vi "charge amplifier.vi"() -> ()   [LabVIEW 2020]
uses:
  <vilib>/Instr/_visa.llb/VISA Configure Serial Port (Instr).vi
panel:
  out "LED CH 4":bool
  out "LED CH 3":bool
  out "LED CH 2":bool
  out "LED CH 1":bool
  in  "CHANNEL 4":bool
  in  "CHANNEL 3":bool
  in  "CHANNEL 2":bool
  in  "CHANNEL 1":bool
  out "Array":bool[](array[boolean])
  in  "ENABLE":bool
  in  "stop":bool
  in  "VISA resource (Arduino)":refnum<visa-resource-name>
  in  "Write":string
  in  "GA2 7":bool
  in  "GA2 6":bool
  in  "GA2 5":bool
  in  "GA2 4":bool
  in  "GA2 3":bool
  in  "GA2 2":bool
  in  "GA2 1":bool
  in  "GA2 0":bool
  in  "GA1 7":bool
  in  "GA1 6":bool
  in  "GA1 5":bool
  in  "GA1 4":bool
  in  "GA1 3":bool
  in  "GA1 2":bool
  in  "GA1 1":bool
  in  "GA1 0":bool
  in  "MUX2 7":bool
  in  "MUX2 6":bool
  in  "MUX2 5":bool
  in  "MUX2 4":bool
  in  "MUX2 3":bool
  in  "MUX2 2":bool
  in  "MUX2 1":bool
  in  "MUX2 0":bool
  in  "MUX1 7":bool
  in  "MUX1 6":bool
  in  "MUX1 5":bool
  in  "MUX1 4":bool
  in  "MUX1 3":bool
  in  "MUX1 2":bool
  in  "MUX1 1":bool
  in  "MUX1 0":bool
  in  "EM2 0":bool
  in  "EM2 1":bool
  in  "EM1 0":bool
  in  "EM1 1":bool
  # "EM1"
  # "EM2"
  # "MUX1"
  # "MUX2"
  # "GAIN1"
  # "GAIN1"
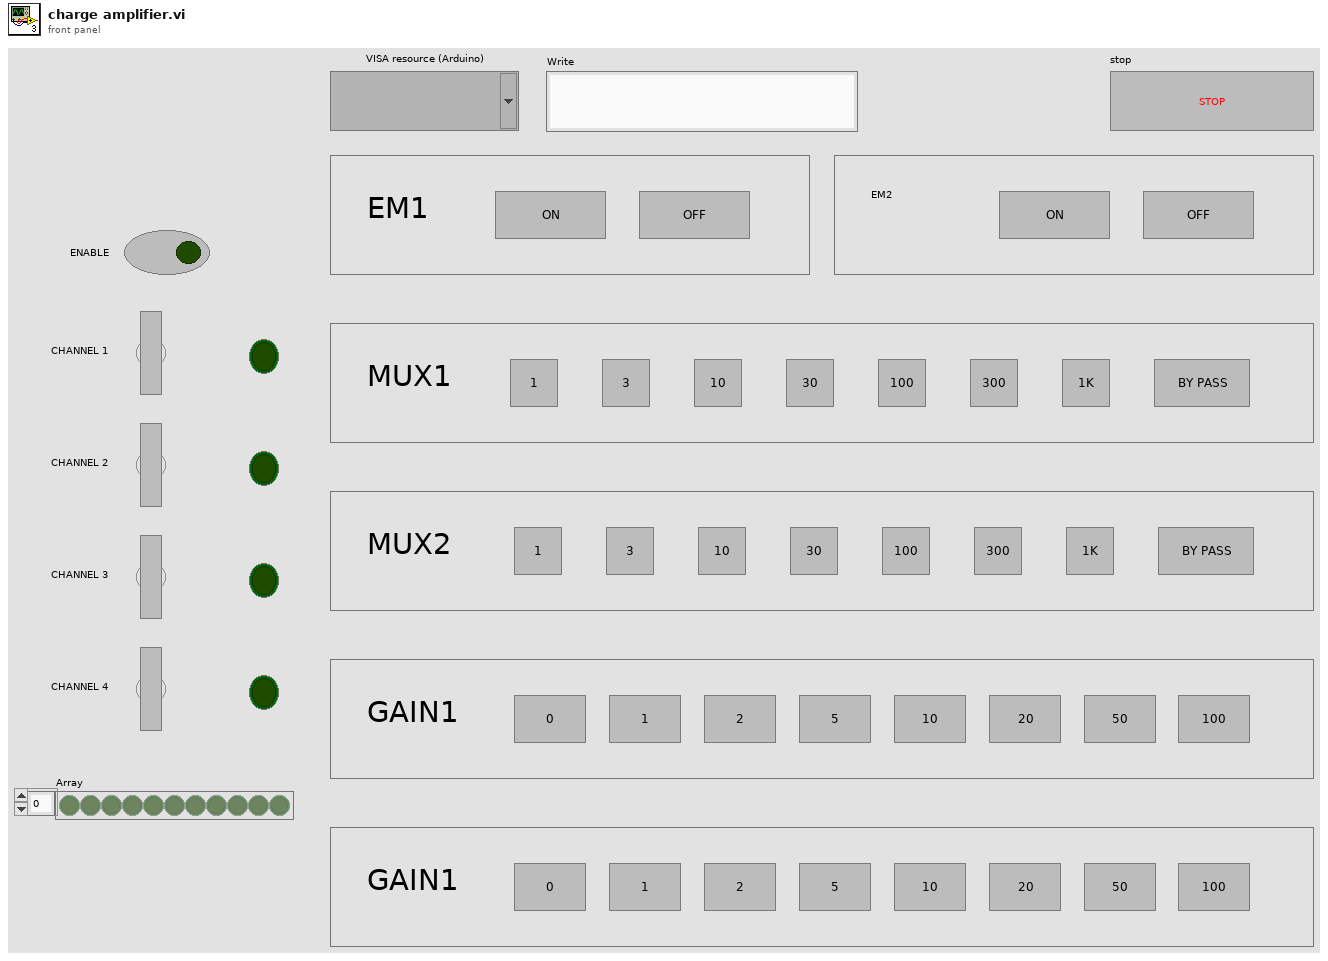
[diagram p1: front panel]
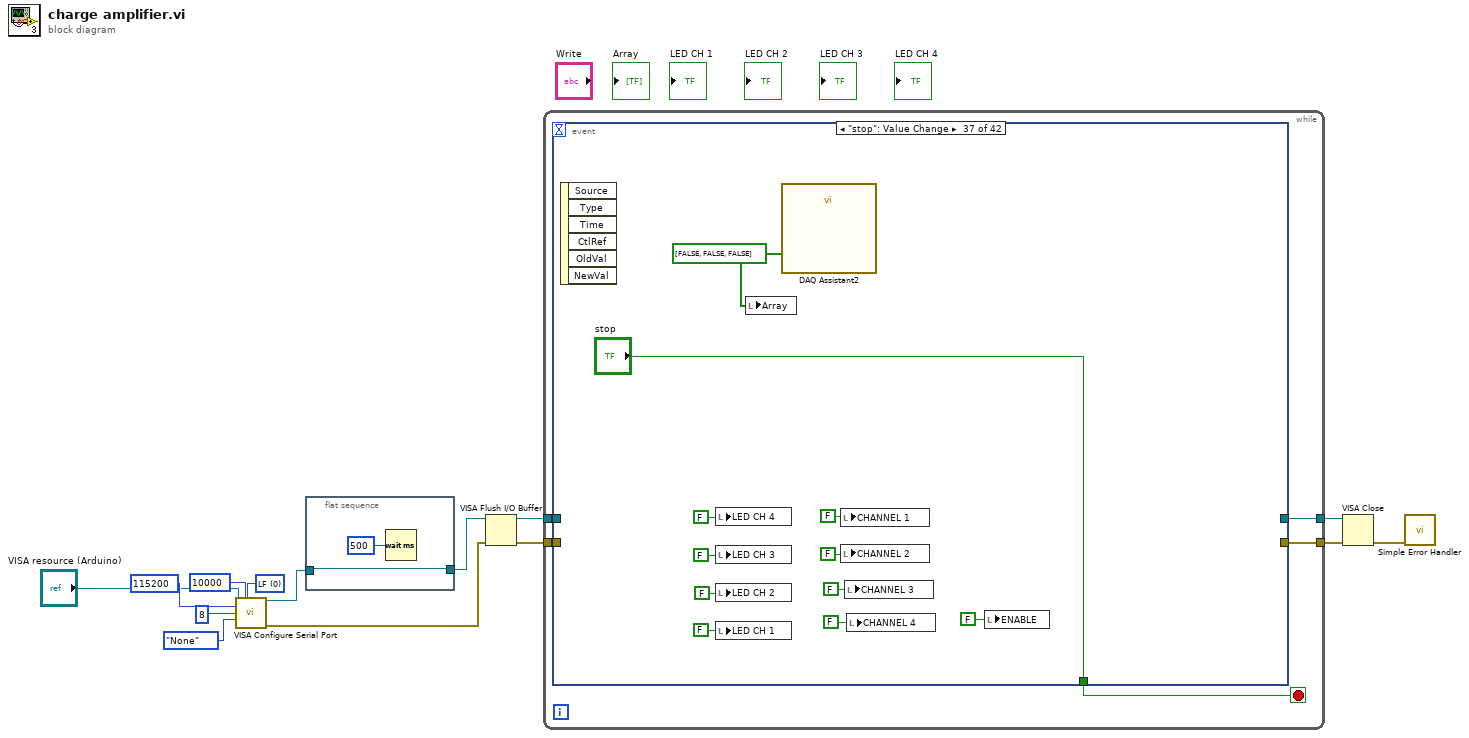
[diagram p0: block diagram]
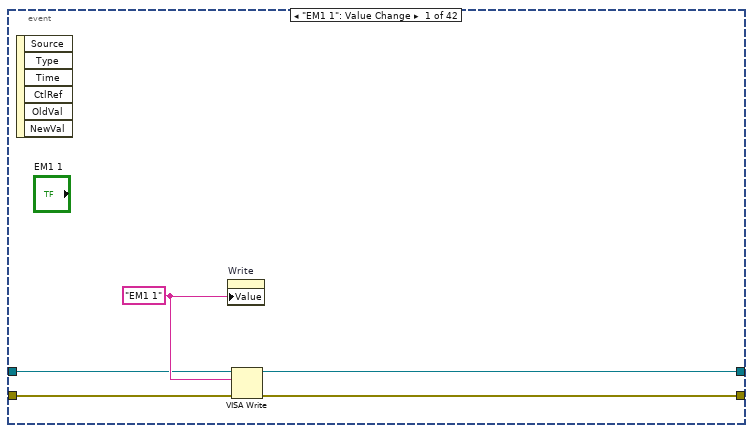
[diagram p2: hidden frame]
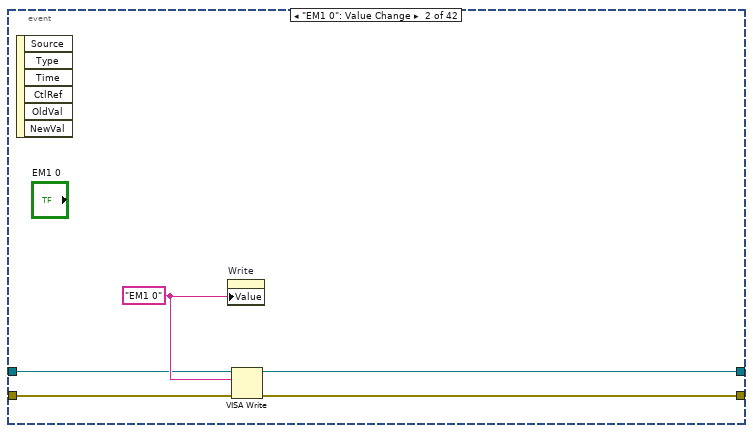
[diagram p3: hidden frame]
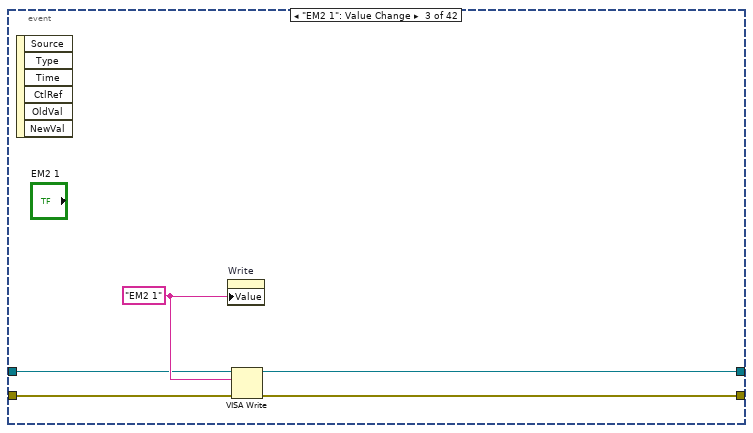
[diagram p4: hidden frame]
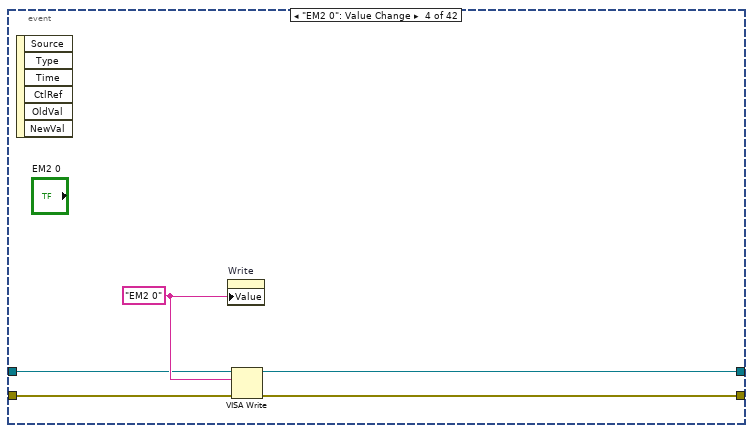
[diagram p5: hidden frame]
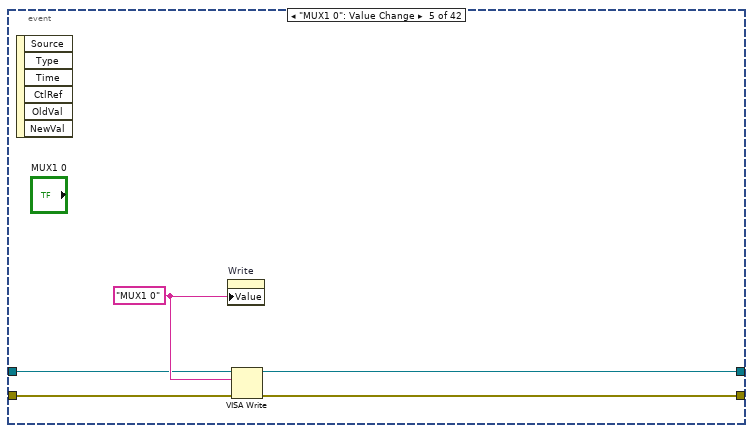
[diagram p6: hidden frame]
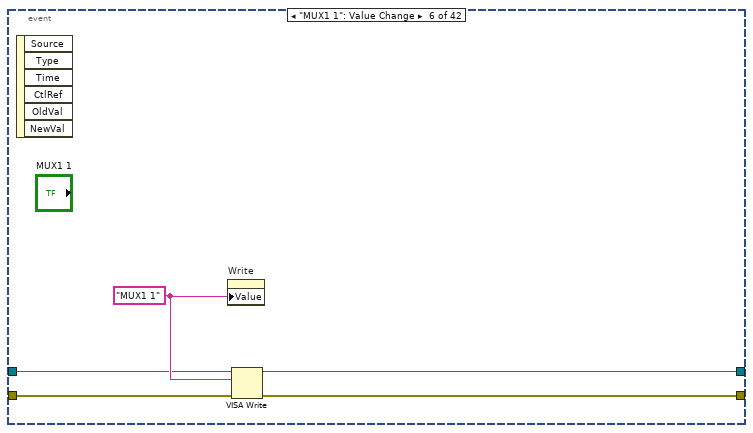
[diagram p7: hidden frame]
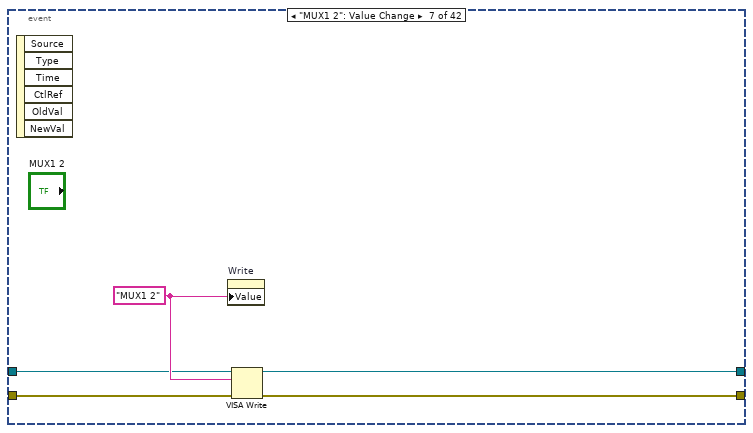
[diagram p8: hidden frame]
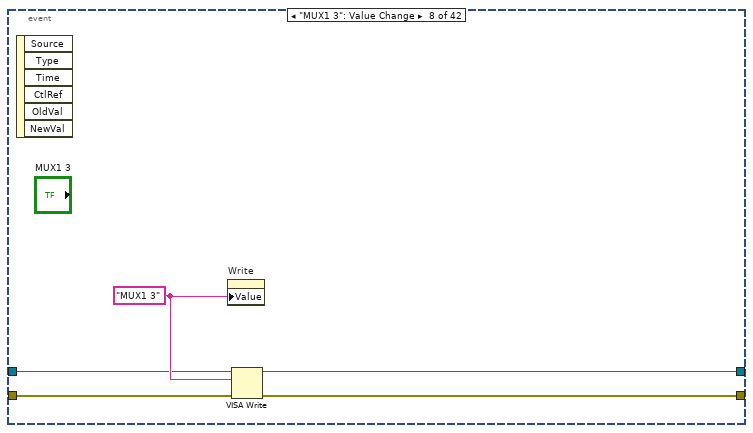
[diagram p9: hidden frame]
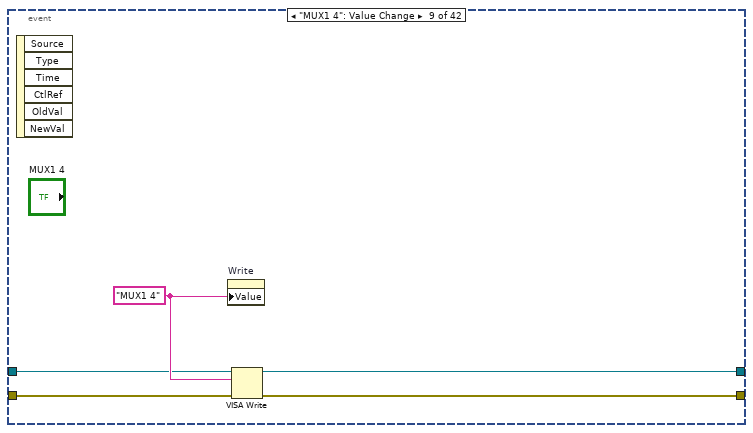
[diagram p10: hidden frame]
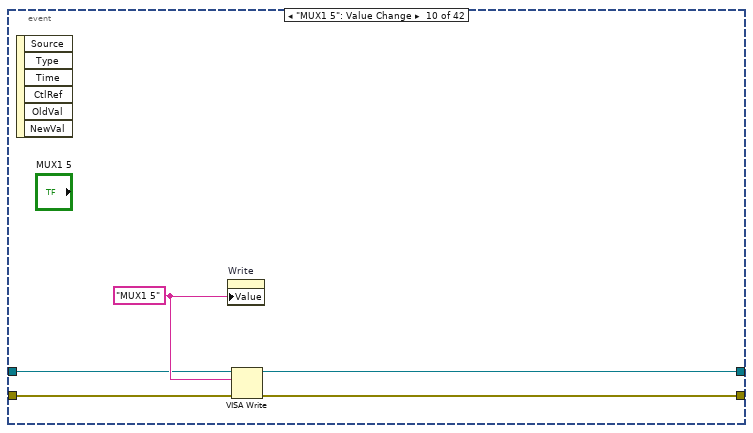
[diagram p11: hidden frame]
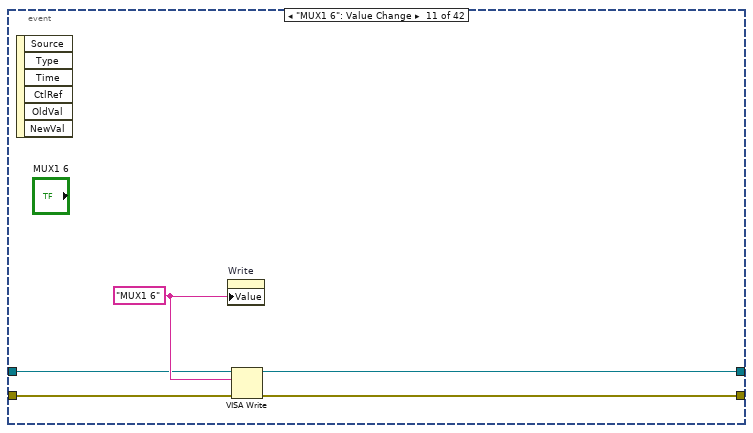
[diagram p12: hidden frame]
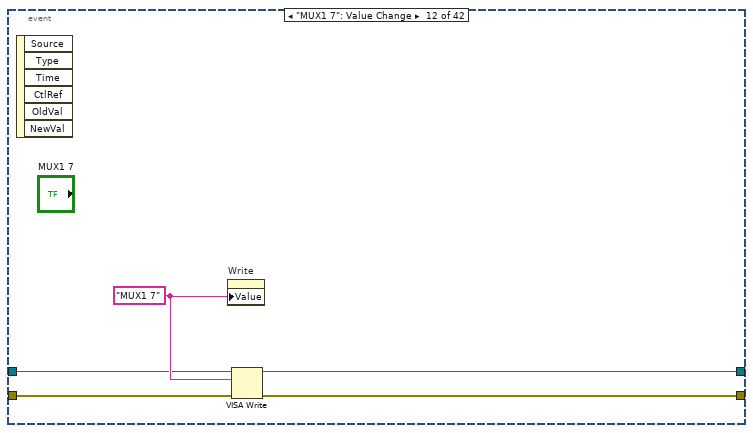
[diagram p13: hidden frame]
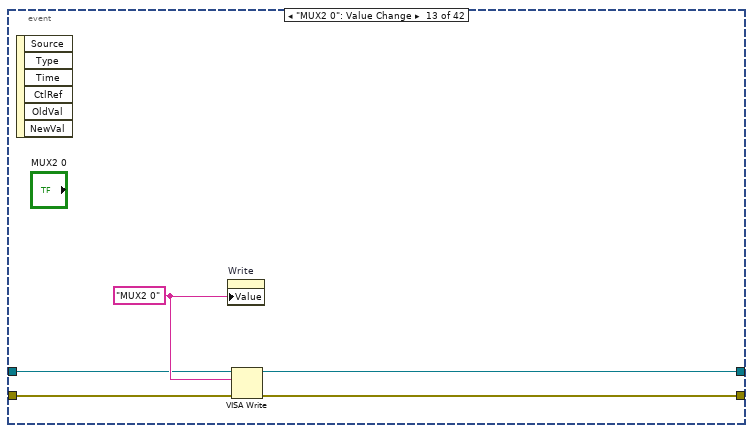
[diagram p14: hidden frame]
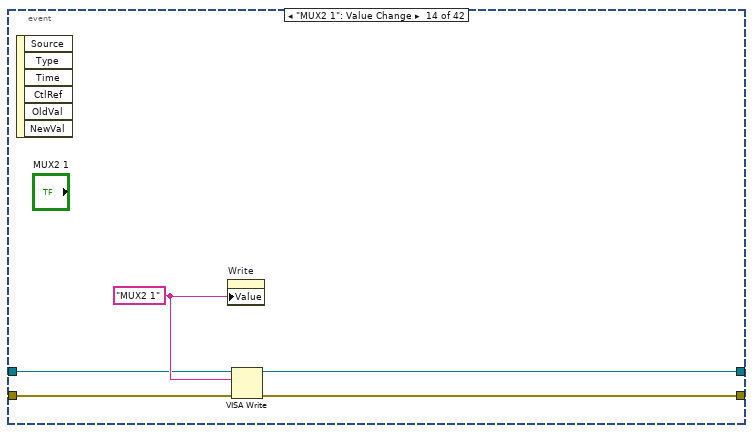
[diagram p15: hidden frame]
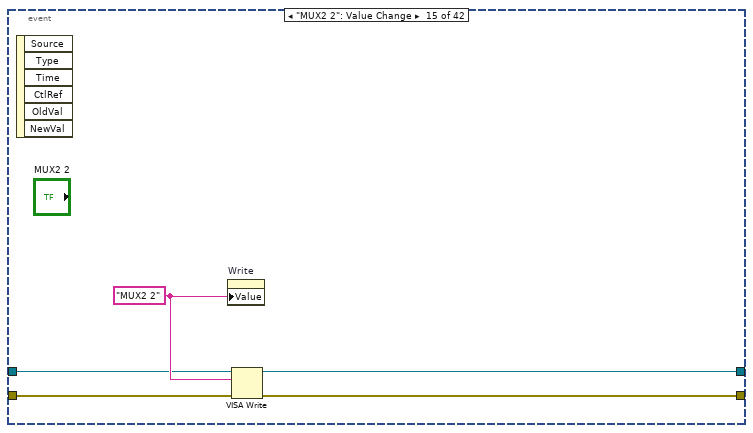
[diagram p16: hidden frame]
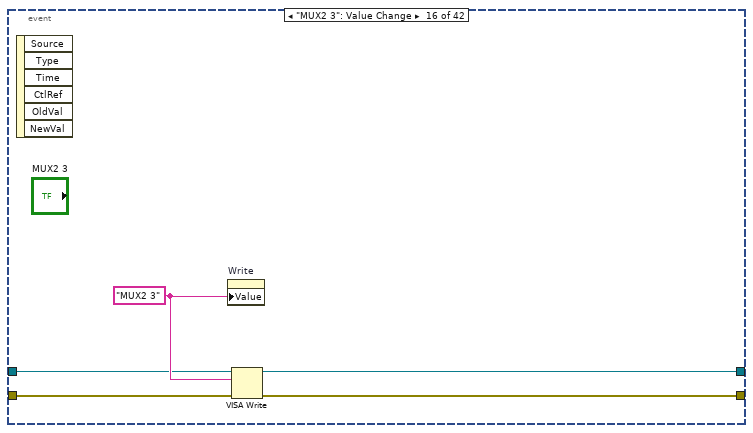
[diagram p17: hidden frame]
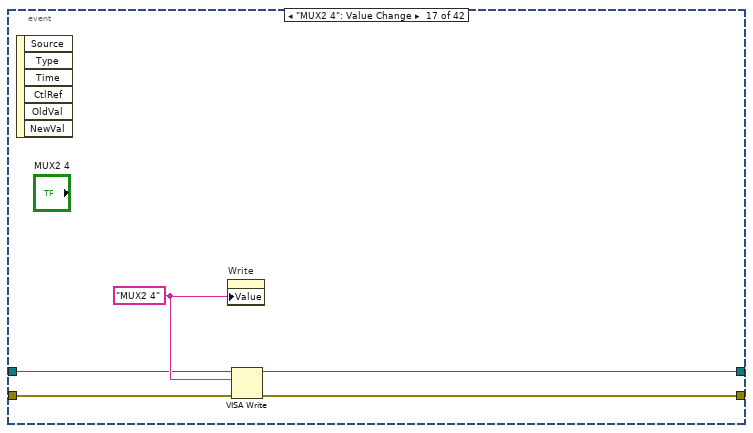
[diagram p18: hidden frame]
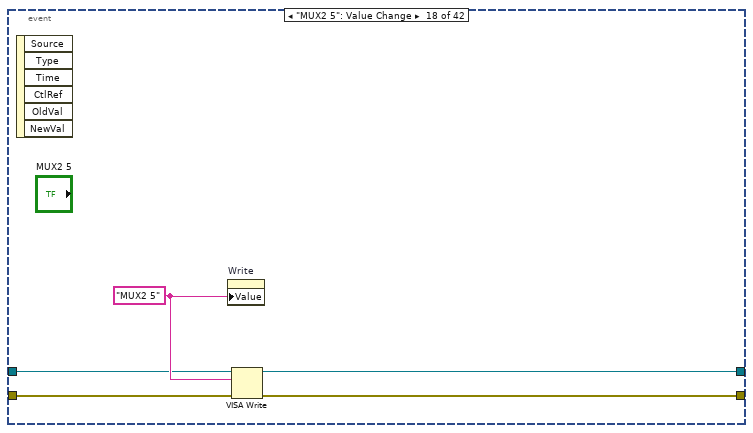
[diagram p19: hidden frame]
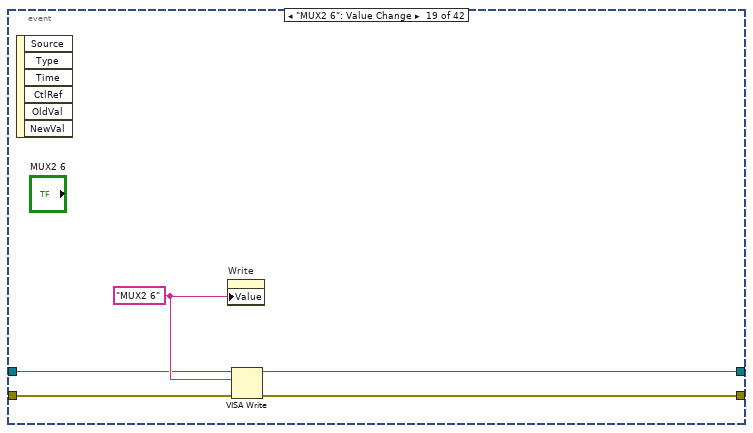
[diagram p20: hidden frame]
diagram:
  w11 = u16 0 items=["LF"]
  n1 = call-poly "VISA Configure Serial Port"("VISA resource name"="VISA resource (Arduino)", "timeout (10sec)"=u32 10000, "termination char\n(0xA = '\\n' = LF)"=w11, "baud rate (9600)"=u32 115200, "data bits (8)"=u16 8, "parity (0:none)"=enum16{"None", "Odd", "Even", "Mark", "Space"}."None") -> ("VISA resource name out"=w7:refnum<visa-resource-name>, "error out"=w5:errorcluster)  [unwired: 8 in]
  n2 = flat-sequence {
    tunnel: [w15] -> w6
    tunnel: w7 -> [w15]
    frame #0 {
      n3 = Wait (ms)(milliseconds to wait=u32 500 ("대기 시간(ms)")) -> ()  [unwired: 1 out]
    }
  }
  n4 = VISA Flush I/O Buffer(VISA resource name=w6, error in (no error)=w5) -> (VISA resource name out=w3:refnum<visa-resource-name>, error out=w2:errorcluster)  [unwired: 1 in]
  n5 = while {
    tunnel: w3 -> [w21]
    tunnel: w2 -> [w20]
    tunnel: [w19] -> w14
    tunnel: [w18] -> w13
    stop <- w17 stop-if-true
    n6 = event shown="[36] \"stop\": Value Change" {
      selector: _ -> [_ _ _ _ _ _ _ _ _ _ _ _ _ _ _ _ _ _ _ _ _ _ _ _ _ _ _ _ _ _ _ _ _ _ _ _ _ _ _ _ _ _]
      dyn-events: _ -> [_ _ _ _ _ _ _ _ _ _ _ _ _ _ _ _ _ _ _ _ _ _ _ _ _ _ _ _ _ _ _ _ _ _ _ _ _ _ _ _ _ _]
      timeout: _ -> [_ _ _ _ _ _ _ _ _ _ _ _ _ _ _ _ _ _ _ _ _ _ _ _ _ _ _ _ _ _ _ _ _ _ _ _ _ _ _ _ _ _]
      tunnel: w21 -> [w25 w30 w35 w40 w45 w50 w55 w60 w65 w70 w75 w80 w85 w90 w95 w100 w105 w110 w115 w120 w125 w130 w135 w140 w145 w150 w155 w160 w165 w170 w175 w180 w185 w190 w195 w200 _ _ _ _ _ _]
      tunnel: w20 -> [w24 w29 w34 w39 w44 w49 w54 w59 w64 w69 w74 w79 w84 w89 w94 w99 w104 w109 w114 w119 w124 w129 w134 w139 w144 w149 w154 w159 w164 w169 w174 w179 w184 w189 w194 w199 _ _ _ _ _ _]
      tunnel: [w23 w28 w33 w38 w43 w48 w53 w58 w63 w68 w73 w78 w83 w88 w93 w98 w103 w108 w113 w118 w123 w128 w133 w138 w143 w148 w153 w158 w163 w168 w173 w178 w183 w188 w193 w198 _ _ _ _ _ _] -> w19
      tunnel: [w22 w27 w32 w37 w42 w47 w52 w57 w62 w67 w72 w77 w82 w87 w92 w97 w102 w107 w112 w117 w122 w127 w132 w137 w142 w147 w152 w157 w162 w167 w172 w177 w182 w187 w192 w197 _ _ _ _ _ _] -> w18
      tunnel: [_ _ _ _ _ _ _ _ _ _ _ _ _ _ _ _ _ _ _ _ _ _ _ _ _ _ _ _ _ _ _ _ _ _ _ _ "stop" _ _ _ _ _] -> w17
      event "EM1 1": Value Change {
        w26 = "EM1 1" ("Write")
        n7 = event-data() -> ()  [unwired: 1 in, 6 out]
        n8 = property on="Write" class="Str"("Value"=w26) -> ()  [unwired: 2 in, 2 out]
        n9 = VISA Write(VISA resource name=w25, write buffer=w26, error in (no error)=w24) -> (VISA resource name out=w23:refnum<visa-resource-name>, error out=w22:errorcluster)  [unwired: 1 out]
      }
      event "EM1 0": Value Change {
        w31 = "EM1 0" ("Write")
        n10 = event-data() -> ()  [unwired: 1 in, 6 out]
        n11 = property on="Write" class="Str"("Value"=w31) -> ()  [unwired: 2 in, 2 out]
        n12 = VISA Write(VISA resource name=w30, write buffer=w31, error in (no error)=w29) -> (VISA resource name out=w28:refnum<visa-resource-name>, error out=w27:errorcluster)  [unwired: 1 out]
      }
      event "EM2 1": Value Change {
        w36 = "EM2 1" ("Write")
        n13 = event-data() -> ()  [unwired: 1 in, 6 out]
        n14 = property on="Write" class="Str"("Value"=w36) -> ()  [unwired: 2 in, 2 out]
        n15 = VISA Write(VISA resource name=w35, write buffer=w36, error in (no error)=w34) -> (VISA resource name out=w33:refnum<visa-resource-name>, error out=w32:errorcluster)  [unwired: 1 out]
      }
      event "EM2 0": Value Change {
        w41 = "EM2 0" ("Write")
        n16 = event-data() -> ()  [unwired: 1 in, 6 out]
        n17 = property on="Write" class="Str"("Value"=w41) -> ()  [unwired: 2 in, 2 out]
        n18 = VISA Write(VISA resource name=w40, write buffer=w41, error in (no error)=w39) -> (VISA resource name out=w38:refnum<visa-resource-name>, error out=w37:errorcluster)  [unwired: 1 out]
      }
      event "MUX1 0": Value Change {
        w46 = "MUX1 0" ("Write")
        n19 = event-data() -> ()  [unwired: 1 in, 6 out]
        n20 = property on="Write" class="Str"("Value"=w46) -> ()  [unwired: 2 in, 2 out]
        n21 = VISA Write(VISA resource name=w45, write buffer=w46, error in (no error)=w44) -> (VISA resource name out=w43:refnum<visa-resource-name>, error out=w42:errorcluster)  [unwired: 1 out]
      }
      event "MUX1 1": Value Change {
        w51 = "MUX1 1" ("Write")
        n22 = event-data() -> ()  [unwired: 1 in, 6 out]
        n23 = property on="Write" class="Str"("Value"=w51) -> ()  [unwired: 2 in, 2 out]
        n24 = VISA Write(VISA resource name=w50, write buffer=w51, error in (no error)=w49) -> (VISA resource name out=w48:refnum<visa-resource-name>, error out=w47:errorcluster)  [unwired: 1 out]
      }
      event "MUX1 2": Value Change {
        w56 = "MUX1 2" ("Write")
        n25 = event-data() -> ()  [unwired: 1 in, 6 out]
        n26 = property on="Write" class="Str"("Value"=w56) -> ()  [unwired: 2 in, 2 out]
        n27 = VISA Write(VISA resource name=w55, write buffer=w56, error in (no error)=w54) -> (VISA resource name out=w53:refnum<visa-resource-name>, error out=w52:errorcluster)  [unwired: 1 out]
      }
      event "MUX1 3": Value Change {
        w61 = "MUX1 3" ("Write")
        n28 = event-data() -> ()  [unwired: 1 in, 6 out]
        n29 = property on="Write" class="Str"("Value"=w61) -> ()  [unwired: 2 in, 2 out]
        n30 = VISA Write(VISA resource name=w60, write buffer=w61, error in (no error)=w59) -> (VISA resource name out=w58:refnum<visa-resource-name>, error out=w57:errorcluster)  [unwired: 1 out]
      }
      event "MUX1 4": Value Change {
        w66 = "MUX1 4" ("Write")
        n31 = event-data() -> ()  [unwired: 1 in, 6 out]
        n32 = property on="Write" class="Str"("Value"=w66) -> ()  [unwired: 2 in, 2 out]
        n33 = VISA Write(VISA resource name=w65, write buffer=w66, error in (no error)=w64) -> (VISA resource name out=w63:refnum<visa-resource-name>, error out=w62:errorcluster)  [unwired: 1 out]
      }
      event "MUX1 5": Value Change {
        w71 = "MUX1 5" ("Write")
        n34 = event-data() -> ()  [unwired: 1 in, 6 out]
        n35 = property on="Write" class="Str"("Value"=w71) -> ()  [unwired: 2 in, 2 out]
        n36 = VISA Write(VISA resource name=w70, write buffer=w71, error in (no error)=w69) -> (VISA resource name out=w68:refnum<visa-resource-name>, error out=w67:errorcluster)  [unwired: 1 out]
      }
      event "MUX1 6": Value Change {
        w76 = "MUX1 6" ("Write")
        n37 = event-data() -> ()  [unwired: 1 in, 6 out]
        n38 = property on="Write" class="Str"("Value"=w76) -> ()  [unwired: 2 in, 2 out]
        n39 = VISA Write(VISA resource name=w75, write buffer=w76, error in (no error)=w74) -> (VISA resource name out=w73:refnum<visa-resource-name>, error out=w72:errorcluster)  [unwired: 1 out]
      }
      event "MUX1 7": Value Change {
        w81 = "MUX1 7" ("Write")
        n40 = event-data() -> ()  [unwired: 1 in, 6 out]
        n41 = property on="Write" class="Str"("Value"=w81) -> ()  [unwired: 2 in, 2 out]
        n42 = VISA Write(VISA resource name=w80, write buffer=w81, error in (no error)=w79) -> (VISA resource name out=w78:refnum<visa-resource-name>, error out=w77:errorcluster)  [unwired: 1 out]
      }
      event "MUX2 0": Value Change {
        w86 = "MUX2 0" ("Write")
        n43 = event-data() -> ()  [unwired: 1 in, 6 out]
        n44 = property on="Write" class="Str"("Value"=w86) -> ()  [unwired: 2 in, 2 out]
        n45 = VISA Write(VISA resource name=w85, write buffer=w86, error in (no error)=w84) -> (VISA resource name out=w83:refnum<visa-resource-name>, error out=w82:errorcluster)  [unwired: 1 out]
      }
      event "MUX2 1": Value Change {
        w91 = "MUX2 1" ("Write")
        n46 = event-data() -> ()  [unwired: 1 in, 6 out]
        n47 = property on="Write" class="Str"("Value"=w91) -> ()  [unwired: 2 in, 2 out]
        n48 = VISA Write(VISA resource name=w90, write buffer=w91, error in (no error)=w89) -> (VISA resource name out=w88:refnum<visa-resource-name>, error out=w87:errorcluster)  [unwired: 1 out]
      }
      event "MUX2 2": Value Change {
        w96 = "MUX2 2" ("Write")
        n49 = event-data() -> ()  [unwired: 1 in, 6 out]
        n50 = property on="Write" class="Str"("Value"=w96) -> ()  [unwired: 2 in, 2 out]
        n51 = VISA Write(VISA resource name=w95, write buffer=w96, error in (no error)=w94) -> (VISA resource name out=w93:refnum<visa-resource-name>, error out=w92:errorcluster)  [unwired: 1 out]
      }
      event "MUX2 3": Value Change {
        w101 = "MUX2 3" ("Write")
        n52 = event-data() -> ()  [unwired: 1 in, 6 out]
        n53 = property on="Write" class="Str"("Value"=w101) -> ()  [unwired: 2 in, 2 out]
        n54 = VISA Write(VISA resource name=w100, write buffer=w101, error in (no error)=w99) -> (VISA resource name out=w98:refnum<visa-resource-name>, error out=w97:errorcluster)  [unwired: 1 out]
      }
      event "MUX2 4": Value Change {
        w106 = "MUX2 4" ("Write")
        n55 = event-data() -> ()  [unwired: 1 in, 6 out]
        n56 = property on="Write" class="Str"("Value"=w106) -> ()  [unwired: 2 in, 2 out]
        n57 = VISA Write(VISA resource name=w105, write buffer=w106, error in (no error)=w104) -> (VISA resource name out=w103:refnum<visa-resource-name>, error out=w102:errorcluster)  [unwired: 1 out]
      }
      event "MUX2 5": Value Change {
        w111 = "MUX2 5" ("Write")
        n58 = event-data() -> ()  [unwired: 1 in, 6 out]
        n59 = property on="Write" class="Str"("Value"=w111) -> ()  [unwired: 2 in, 2 out]
        n60 = VISA Write(VISA resource name=w110, write buffer=w111, error in (no error)=w109) -> (VISA resource name out=w108:refnum<visa-resource-name>, error out=w107:errorcluster)  [unwired: 1 out]
      }
      event "MUX2 6": Value Change {
        w116 = "MUX2 6" ("Write")
        n61 = event-data() -> ()  [unwired: 1 in, 6 out]
        n62 = property on="Write" class="Str"("Value"=w116) -> ()  [unwired: 2 in, 2 out]
        n63 = VISA Write(VISA resource name=w115, write buffer=w116, error in (no error)=w114) -> (VISA resource name out=w113:refnum<visa-resource-name>, error out=w112:errorcluster)  [unwired: 1 out]
      }
      event "MUX2 7": Value Change {
        w121 = "MUX2 7" ("Write")
        n64 = event-data() -> ()  [unwired: 1 in, 6 out]
        n65 = property on="Write" class="Str"("Value"=w121) -> ()  [unwired: 2 in, 2 out]
        n66 = VISA Write(VISA resource name=w120, write buffer=w121, error in (no error)=w119) -> (VISA resource name out=w118:refnum<visa-resource-name>, error out=w117:errorcluster)  [unwired: 1 out]
      }
      event "GA1 0": Value Change {
        w126 = "GA1 0" ("Write")
        n67 = event-data() -> ()  [unwired: 1 in, 6 out]
        n68 = property on="Write" class="Str"("Value"=w126) -> ()  [unwired: 2 in, 2 out]
        n69 = VISA Write(VISA resource name=w125, write buffer=w126, error in (no error)=w124) -> (VISA resource name out=w123:refnum<visa-resource-name>, error out=w122:errorcluster)  [unwired: 1 out]
      }
      event "GA1 1": Value Change {
        w131 = "GA1 1" ("Write")
        n70 = event-data() -> ()  [unwired: 1 in, 6 out]
        n71 = property on="Write" class="Str"("Value"=w131) -> ()  [unwired: 2 in, 2 out]
        n72 = VISA Write(VISA resource name=w130, write buffer=w131, error in (no error)=w129) -> (VISA resource name out=w128:refnum<visa-resource-name>, error out=w127:errorcluster)  [unwired: 1 out]
      }
      event "GA1 2": Value Change {
        w136 = "GA1 2" ("Write")
        n73 = event-data() -> ()  [unwired: 1 in, 6 out]
        n74 = property on="Write" class="Str"("Value"=w136) -> ()  [unwired: 2 in, 2 out]
        n75 = VISA Write(VISA resource name=w135, write buffer=w136, error in (no error)=w134) -> (VISA resource name out=w133:refnum<visa-resource-name>, error out=w132:errorcluster)  [unwired: 1 out]
      }
      event "GA1 3": Value Change {
        w141 = "GA1 3" ("Write")
        n76 = event-data() -> ()  [unwired: 1 in, 6 out]
        n77 = property on="Write" class="Str"("Value"=w141) -> ()  [unwired: 2 in, 2 out]
        n78 = VISA Write(VISA resource name=w140, write buffer=w141, error in (no error)=w139) -> (VISA resource name out=w138:refnum<visa-resource-name>, error out=w137:errorcluster)  [unwired: 1 out]
      }
      event "GA1 4": Value Change {
        w146 = "GA1 4" ("Write")
        n79 = event-data() -> ()  [unwired: 1 in, 6 out]
        n80 = property on="Write" class="Str"("Value"=w146) -> ()  [unwired: 2 in, 2 out]
        n81 = VISA Write(VISA resource name=w145, write buffer=w146, error in (no error)=w144) -> (VISA resource name out=w143:refnum<visa-resource-name>, error out=w142:errorcluster)  [unwired: 1 out]
      }
      event "GA1 5": Value Change {
        w151 = "GA1 5" ("Write")
        n82 = event-data() -> ()  [unwired: 1 in, 6 out]
        n83 = property on="Write" class="Str"("Value"=w151) -> ()  [unwired: 2 in, 2 out]
        n84 = VISA Write(VISA resource name=w150, write buffer=w151, error in (no error)=w149) -> (VISA resource name out=w148:refnum<visa-resource-name>, error out=w147:errorcluster)  [unwired: 1 out]
      }
      event "GA1 6": Value Change {
        w156 = "GA1 6" ("Write")
        n85 = event-data() -> ()  [unwired: 1 in, 6 out]
        n86 = property on="Write" class="Str"("Value"=w156) -> ()  [unwired: 2 in, 2 out]
        n87 = VISA Write(VISA resource name=w155, write buffer=w156, error in (no error)=w154) -> (VISA resource name out=w153:refnum<visa-resource-name>, error out=w152:errorcluster)  [unwired: 1 out]
      }
      event "GA1 7": Value Change {
        w161 = "GA1 7" ("Write")
        n88 = event-data() -> ()  [unwired: 1 in, 6 out]
        n89 = property on="Write" class="Str"("Value"=w161) -> ()  [unwired: 2 in, 2 out]
        n90 = VISA Write(VISA resource name=w160, write buffer=w161, error in (no error)=w159) -> (VISA resource name out=w158:refnum<visa-resource-name>, error out=w157:errorcluster)  [unwired: 1 out]
      }
      event "GA2 0": Value Change {
        w166 = "GA2 0" ("Write")
        n91 = event-data() -> ()  [unwired: 1 in, 6 out]
        n92 = property on="Write" class="Str"("Value"=w166) -> ()  [unwired: 2 in, 2 out]
        n93 = VISA Write(VISA resource name=w165, write buffer=w166, error in (no error)=w164) -> (VISA resource name out=w163:refnum<visa-resource-name>, error out=w162:errorcluster)  [unwired: 1 out]
      }
      event "GA2 1": Value Change {
        w171 = "GA2 1" ("Write")
        n94 = event-data() -> ()  [unwired: 1 in, 6 out]
        n95 = property on="Write" class="Str"("Value"=w171) -> ()  [unwired: 2 in, 2 out]
        n96 = VISA Write(VISA resource name=w170, write buffer=w171, error in (no error)=w169) -> (VISA resource name out=w168:refnum<visa-resource-name>, error out=w167:errorcluster)  [unwired: 1 out]
      }
      event "GA2 2": Value Change {
        w176 = "GA2 2" ("Write")
        n97 = event-data() -> ()  [unwired: 1 in, 6 out]
        n98 = property on="Write" class="Str"("Value"=w176) -> ()  [unwired: 2 in, 2 out]
        n99 = VISA Write(VISA resource name=w175, write buffer=w176, error in (no error)=w174) -> (VISA resource name out=w173:refnum<visa-resource-name>, error out=w172:errorcluster)  [unwired: 1 out]
      }
      event "GA2 3": Value Change {
        w181 = "GA2 3" ("Write")
        n100 = event-data() -> ()  [unwired: 1 in, 6 out]
        n101 = property on="Write" class="Str"("Value"=w181) -> ()  [unwired: 2 in, 2 out]
        n102 = VISA Write(VISA resource name=w180, write buffer=w181, error in (no error)=w179) -> (VISA resource name out=w178:refnum<visa-resource-name>, error out=w177:errorcluster)  [unwired: 1 out]
      }
      event "GA2 4": Value Change {
        w186 = "GA2 4" ("Write")
        n103 = event-data() -> ()  [unwired: 1 in, 6 out]
        n104 = property on="Write" class="Str"("Value"=w186) -> ()  [unwired: 2 in, 2 out]
        n105 = VISA Write(VISA resource name=w185, write buffer=w186, error in (no error)=w184) -> (VISA resource name out=w183:refnum<visa-resource-name>, error out=w182:errorcluster)  [unwired: 1 out]
      }
      event "GA2 5": Value Change {
        w191 = "GA2 5" ("Write")
        n106 = event-data() -> ()  [unwired: 1 in, 6 out]
        n107 = property on="Write" class="Str"("Value"=w191) -> ()  [unwired: 2 in, 2 out]
        n108 = VISA Write(VISA resource name=w190, write buffer=w191, error in (no error)=w189) -> (VISA resource name out=w188:refnum<visa-resource-name>, error out=w187:errorcluster)  [unwired: 1 out]
      }
      event "GA2 6": Value Change {
        w196 = "GA2 6" ("Write")
        n109 = event-data() -> ()  [unwired: 1 in, 6 out]
        n110 = property on="Write" class="Str"("Value"=w196) -> ()  [unwired: 2 in, 2 out]
        n111 = VISA Write(VISA resource name=w195, write buffer=w196, error in (no error)=w194) -> (VISA resource name out=w193:refnum<visa-resource-name>, error out=w192:errorcluster)  [unwired: 1 out]
      }
      event "GA2 7": Value Change {
        w201 = "GA2 7" ("Write")
        n112 = event-data() -> ()  [unwired: 1 in, 6 out]
        n113 = property on="Write" class="Str"("Value"=w201) -> ()  [unwired: 2 in, 2 out]
        n114 = VISA Write(VISA resource name=w200, write buffer=w201, error in (no error)=w199) -> (VISA resource name out=w198:refnum<visa-resource-name>, error out=w197:errorcluster)  [unwired: 1 out]
      }
      event "stop": Value Change {
        w202 = bool[] [FALSE, FALSE, FALSE]
        n115 = event-data() -> ()  [unwired: 1 in, 6 out]
        n116 = local write "LED CH 4"(FALSE ("ENABLE")) -> ()
        n117 = local write "LED CH 3"(FALSE ("ENABLE")) -> ()
        n118 = local write "LED CH 2"(FALSE ("ENABLE")) -> ()
        n119 = local write "LED CH 1"(FALSE ("ENABLE")) -> ()
        n120 = local write "Array"(w202) -> ()
        n121 = call "DAQ Assistant2"("data"=w202) -> ()  [unwired: 17 in, 2 out]
        n122 = local write "CHANNEL 1"(FALSE ("ENABLE")) -> ()
        n123 = local write "CHANNEL 2"(FALSE ("ENABLE")) -> ()
        n124 = local write "CHANNEL 3"(FALSE ("ENABLE")) -> ()
        n125 = local write "CHANNEL 4"(FALSE ("ENABLE")) -> ()
        n126 = local write "ENABLE"(FALSE ("ENABLE")) -> ()
      }
      event "CHANNEL 1": Value Change {
        n127 = event-data() -> ()  [unwired: 1 in, 6 out]
        n128 = local read "ENABLE"() -> (w213:bool)
        n129 = case shown="True" w213 {
          frame False {
          }
          frame True {
            w215 = FALSE ("CHANNEL 4")
            w216 = FALSE ("CHANNEL 3")
            w217 = FALSE ("CHANNEL 2")
            w218 = bool[] [TRUE, FALSE, FALSE]
            n130 = property on="CHANNEL 3" class="Bool (strict)"("Value"=w216) -> ()  [unwired: 2 in, 2 out]
            n131 = property on="CHANNEL 2" class="Bool (strict)"("Value"=w217) -> ()  [unwired: 2 in, 2 out]
            n132 = property on="CHANNEL 4" class="Bool (strict)"("Value"=w215) -> ()  [unwired: 2 in, 2 out]
            n133 = local write "LED CH 1"(TRUE ("LED CH 1")) -> ()
            n134 = local write "LED CH 2"(w217) -> ()
            n135 = local write "LED CH 3"(w216) -> ()
            n136 = local write "LED CH 4"(w215) -> ()
            n137 = local write "Array"(w218) -> ()
            n138 = call "DAQ Assistant3"("data"=w218) -> ()  [unwired: 17 in, 2 out]
          }
        }
      }
      event "CHANNEL 2": Value Change {
        n139 = event-data() -> ()  [unwired: 1 in, 6 out]
        n140 = local read "ENABLE"() -> (w219:bool)
        n141 = case shown="False" w219 {
          frame False {
          }
          frame True {
            w221 = FALSE ("CHANNEL 4")
            w222 = FALSE ("CHANNEL 3")
            w223 = FALSE ("CHANNEL 1")
            w224 = bool[] [TRUE, FALSE, TRUE]
            n142 = property on="CHANNEL 1" class="Bool (strict)"("Value"=w223) -> ()  [unwired: 2 in, 2 out]
            n143 = property on="CHANNEL 3" class="Bool (strict)"("Value"=w222) -> ()  [unwired: 2 in, 2 out]
            n144 = property on="CHANNEL 4" class="Bool (strict)"("Value"=w221) -> ()  [unwired: 2 in, 2 out]
            n145 = local write "LED CH 2"(TRUE ("LED CH 2")) -> ()
            n146 = local write "LED CH 1"(w223) -> ()
            n147 = local write "LED CH 3"(w222) -> ()
            n148 = local write "LED CH 4"(w221) -> ()
            n149 = local write "Array"(w224) -> ()
            n150 = call "DAQ Assistant5"("data"=w224) -> ()  [unwired: 17 in, 2 out]
          }
        }
      }
      event "CHANNEL 3": Value Change {
        n151 = event-data() -> ()  [unwired: 1 in, 6 out]
        n152 = local read "ENABLE"() -> (w225:bool)
        n153 = case shown="False" w225 {
          frame False {
          }
          frame True {
            w229 = FALSE ("CHANNEL 4")
            w228 = FALSE ("CHANNEL 2")
            w227 = FALSE ("CHANNEL 1")
            w230 = bool[] [TRUE, TRUE, FALSE]
            n154 = property on="CHANNEL 1" class="Bool (strict)"("Value"=w227) -> ()  [unwired: 2 in, 2 out]
            n155 = property on="CHANNEL 2" class="Bool (strict)"("Value"=w228) -> ()  [unwired: 2 in, 2 out]
            n156 = property on="CHANNEL 4" class="Bool (strict)"("Value"=w229) -> ()  [unwired: 2 in, 2 out]
            n157 = local write "LED CH 3"(TRUE ("LED CH 3")) -> ()
            n158 = local write "LED CH 1"(w227) -> ()
            n159 = local write "LED CH 2"(w228) -> ()
            n160 = local write "LED CH 4"(w229) -> ()
            n161 = call "DAQ Assistant7"("data"=w230) -> ()  [unwired: 17 in, 2 out]
            n162 = local write "Array"(w230) -> ()
          }
        }
      }
      event "CHANNEL 4": Value Change {
        n163 = event-data() -> ()  [unwired: 1 in, 6 out]
        n164 = local read "ENABLE"() -> (w231:bool)
        n165 = case shown="True" w231 {
          frame False {
          }
          frame True {
            w235 = FALSE ("CHANNEL 3")
            w234 = FALSE ("CHANNEL 2")
            w233 = FALSE ("CHANNEL 1")
            w236 = bool[] [TRUE, TRUE, TRUE]
            n166 = property on="CHANNEL 3" class="Bool (strict)"("Value"=w235) -> ()  [unwired: 2 in, 2 out]
            n167 = property on="CHANNEL 1" class="Bool (strict)"("Value"=w233) -> ()  [unwired: 2 in, 2 out]
            n168 = property on="CHANNEL 2" class="Bool (strict)"("Value"=w234) -> ()  [unwired: 2 in, 2 out]
            n169 = local write "LED CH 1"(w233) -> ()
            n170 = local write "LED CH 2"(w234) -> ()
            n171 = local write "LED CH 3"(w235) -> ()
            n172 = local write "LED CH 4"(TRUE ("LED CH 4")) -> ()
            n173 = call "DAQ Assistant9"("data"=w236) -> ()  [unwired: 17 in, 2 out]
            n174 = local write "Array"(w236) -> ()
          }
        }
      }
      event "ENABLE": Value Change {
        n175 = event-data() -> ()  [unwired: 1 in, 6 out]
        n176 = local read "ENABLE"() -> (w237:bool)
        n177 = case shown="True" w237 {
          frame False {
            w241 = FALSE ("CHANNEL 4")
            w240 = FALSE ("CHANNEL 3")
            w239 = FALSE ("CHANNEL 2")
            w238 = FALSE ("CHANNEL 1")
            w242 = bool[] [FALSE, FALSE, FALSE]
            n178 = property on="CHANNEL 3" class="Bool (strict)"("Value"=w240) -> ()  [unwired: 2 in, 2 out]
            n179 = property on="CHANNEL 1" class="Bool (strict)"("Value"=w238) -> ()  [unwired: 2 in, 2 out]
            n180 = property on="CHANNEL 2" class="Bool (strict)"("Value"=w239) -> ()  [unwired: 2 in, 2 out]
            n181 = property on="CHANNEL 4" class="Bool (strict)"("Value"=w241) -> ()  [unwired: 2 in, 2 out]
            n182 = local write "LED CH 1"(w238) -> ()
            n183 = local write "LED CH 2"(w239) -> ()
            n184 = local write "LED CH 3"(w240) -> ()
            n185 = local write "LED CH 4"(w241) -> ()
            n186 = local write "Array"(w242) -> ()
            n187 = call "DAQ Assistant10"("data"=w242) -> ()  [unwired: 17 in, 2 out]
          }
          frame True {
            w246 = FALSE ("CHANNEL 4")
            w245 = FALSE ("CHANNEL 3")
            w244 = FALSE ("CHANNEL 2")
            w243 = TRUE ("CHANNEL 1")
            w247 = bool[] [TRUE, FALSE, FALSE]
            n188 = property on="CHANNEL 3" class="Bool (strict)"("Value"=w245) -> ()  [unwired: 2 in, 2 out]
            n189 = property on="CHANNEL 1" class="Bool (strict)"("Value"=w243) -> ()  [unwired: 2 in, 2 out]
            n190 = property on="CHANNEL 2" class="Bool (strict)"("Value"=w244) -> ()  [unwired: 2 in, 2 out]
            n191 = property on="CHANNEL 4" class="Bool (strict)"("Value"=w246) -> ()  [unwired: 2 in, 2 out]
            n192 = local write "LED CH 1"(w243) -> ()
            n193 = local write "LED CH 2"(w244) -> ()
            n194 = local write "LED CH 3"(w245) -> ()
            n195 = local write "LED CH 4"(w246) -> ()
            n196 = local write "Array"(w247) -> ()
            n197 = call "DAQ Assistant"("data"=w247) -> ()  [unwired: 17 in, 2 out]
          }
        }
      }
    }
  }
  n198 = VISA Close(VISA resource name=w14, error in (no error)=w13) -> (error out=w1:errorcluster)
  n199 = call <vilib>:"Simple Error Handler.vi"("error in (no error)"=w1) -> ()  [unwired: 4 in, 5 out]
